vi "MeasureAtFreq.vi"(8 "error in (no error)":errorcluster, 10 "Frequency (Hz)":dbl, 11 "PwrMtr_U2k in":refnum<class "PwrMtr_U2k.lvclass">) -> (0 "error out":errorcluster, 2 "Power (dBm)":dbl, 3 "PwrMtr_U2k out":refnum<class "PwrMtr_U2k.lvclass">)   [LabVIEW 2014, in "PwrMtr_U2k.lvclass"]
uses:
  PwrMtr_U2k.lvclass
  PwrMtr_U2k.lvclass/PwrMtr_U2k.ctl
  <instrlib>/Agilent U2000 Series/Public/Data/Low Level/Initiate (Immediate).vi
  <instrlib>/Agilent U2000 Series/Agilent U2000 Series.lvlib
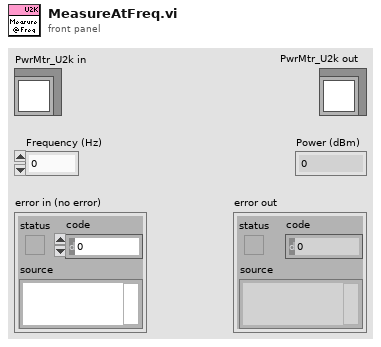
[diagram p1: front panel]
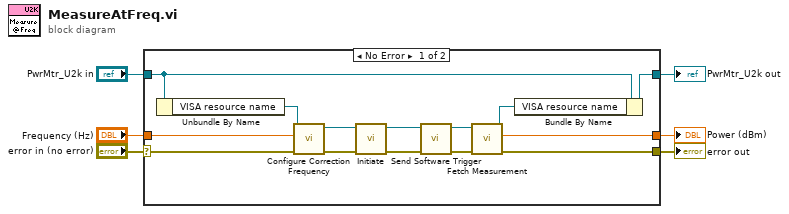
[diagram p0: block diagram]
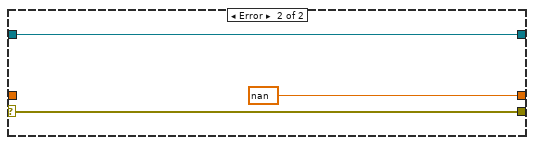
[diagram p2: hidden frame]
diagram:
  n1 = case shown="No Error" "error in (no error)" {
    selector: "error in (no error)" -> [w20 w22]
    tunnel: "Frequency (Hz)" -> [w18 _]
    tunnel: "PwrMtr_U2k in" -> [w16 w23]
    tunnel: [w19 w22] -> w4
    tunnel: [w17 nan ("Amplitude (Cal)")] -> w3
    tunnel: [w15 w23] -> w1
    frame No Error {
      n2 = Unbundle By Name(w16) -> ("VISA resource name"=w14:refnum<visa-resource-name>)
      n3 = call <instrlib>:"Configure Correction Frequency.vi"("error in (no error)"=w20, "Frequency (5E+7 Hz)"=w18, "VISA resource name"=w14) -> ("error out"=w12:errorcluster, "VISA resource name out"=w11:refnum<visa-resource-name>)  [unwired: 7 in]
      n4 = call-poly <instrlib>:"Initiate.vi"("error in (no error)"=w12, "VISA resource name"=w11) -> ("error out"=w10:errorcluster, "VISA resource name out"=w9:refnum<visa-resource-name>)  [unwired: 8 in]
      n5 = call <instrlib>:"Send Software Trigger.vi"("error in (no error)"=w10, "VISA resource name"=w9) -> ("error out"=w8:errorcluster, "VISA resource name out"=w7:refnum<visa-resource-name>)  [unwired: 8 in]
      n6 = call <instrlib>:"Fetch Measurement.vi"("error in (no error)"=w8, "VISA resource name"=w7) -> ("error out"=w19:errorcluster, "Measurement"=w17:dbl, "VISA resource name out"=w13:refnum<visa-resource-name>)  [unwired: 1 in, 6 out]
      n7 = Bundle By Name(cluster=w16, "VISA resource name"=w13) -> (w15:refnum<class "PwrMtr_U2k.lvclass">)
    }
    frame Error {
    }
  }
  "error out" <- w4
  "Power (dBm)" <- w3
  "PwrMtr_U2k out" <- w1
